vi "Breadth-First-Search.vi"(9 "Tag":string, 11 "Tree in":refnum<class "Tree.lvclass">) -> (3 "Tree out":refnum<class "Tree.lvclass">)   [LabVIEW 2022 SP3, in "Tree.lvclass"]
uses:
  Tree.lvclass
  Type Def/Single Level.ctl
  Type Def/Tree Item.ctl
  Tree.lvclass/Tree.ctl
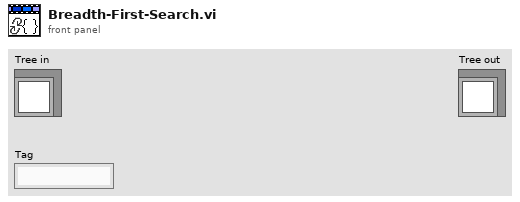
[diagram p1: front panel]
types:
  T1 = typedef "Single Level.ctl" = cluster{"Level Items":T2[]}
  T2 = typedef "Tree Item.ctl" = cluster{"Parent Tag":string, "Tag":string, "Left Cell":string, "Cells Text":string[], "BFS Index":i32[], "Graph Index":i32, "Item Indent":i32}
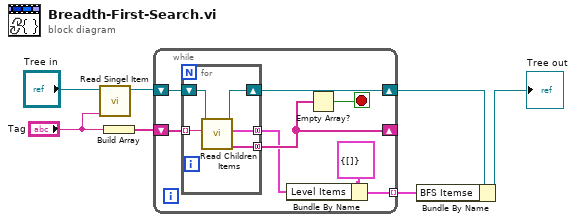
[diagram p0: block diagram]
diagram:
  n1 = call "Read Singel Item.vi"("Tag"="Tag", "Tree in"="Tree in") -> ("Tree out"=w3:refnum<class "Tree.lvclass">)  [unwired: 8 in, 1 out]
  n2 = Build Array("Tag") -> (w7:string[])
  n3 = while {
    shift-right: [w12] -> _
    shift-left: w7 -> [w13]
    shift-right: [w14] -> w6
    shift-left: w3 -> [w15]
    tunnel: [w8] -> w5 mode=indexing
    stop <- w11 stop-if-true
    n4 = for {
      shift-right: [w19] -> w14
      shift-left: w15 -> [w20]
      tunnel: w13 -> [w18] mode=indexing
      tunnel: [w17] -> w9 mode=concatenating
      tunnel: [w16] -> w12 mode=concatenating
      n5 = call "Read Children Items.vi"("Tag In"=w18, "Tree in"=w20) -> ("Children Tag"=w16:string[], "Children Items"=w17:T2[], "Tree out"=w19:refnum<class "Tree.lvclass">)  [unwired: 7 in]
    }
    n6 = Bundle By Name(cluster=T1 {"Level Items"=[]} ("Single Level"), "Level Items"=w9) -> (w8:T1)
    n7 = Empty Array?(array=w12) -> (empty?=w11:bool)
  }
  n8 = Bundle By Name(cluster=w6, "BFS Itemse"=w5) -> (→"Tree out":refnum<class "Tree.lvclass">)
